vi "Remove Logged Cal.vi"(8 "error in (no error)":errorcluster, 11 "array results in":T1) -> (0 "error out":errorcluster, 2 "update results?":bool, 3 "array results out":T1)   [LabVIEW 2020]
uses:
  Controller Loop/Controller Data.ctl
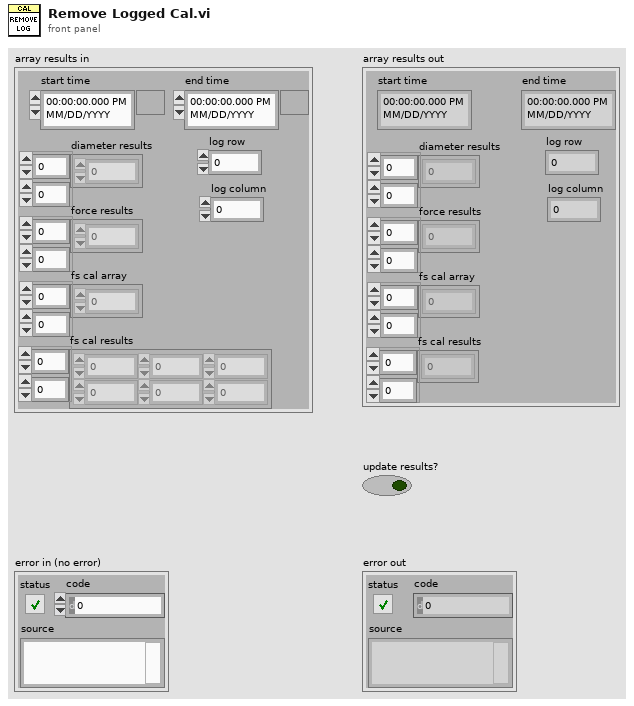
[diagram p1: front panel]
types:
  T1 = typedef "Controller Data.ctl" = cluster{"diameter results":dbl[][], "force results":dbl[][], "fs cal array":dbl[][], "fs cal results":dbl[][], "start time":timestamp, "end time":timestamp, "log row":i32, "log column":i32}
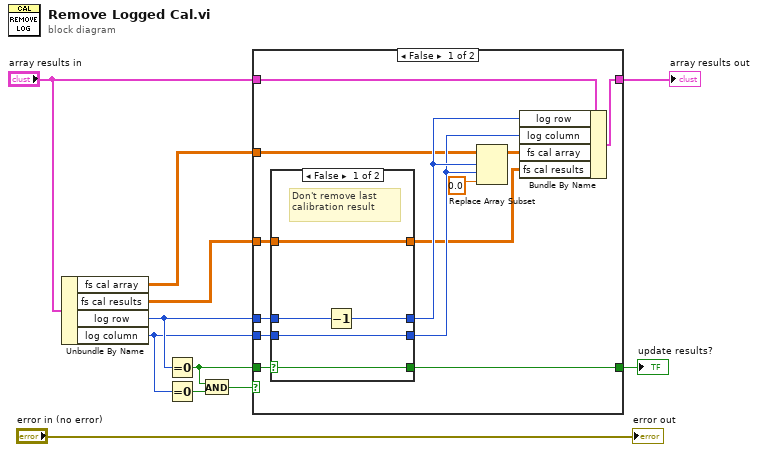
[diagram p0: block diagram]
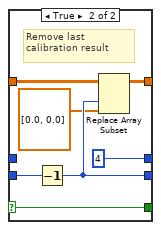
[diagram p2: hidden frame]
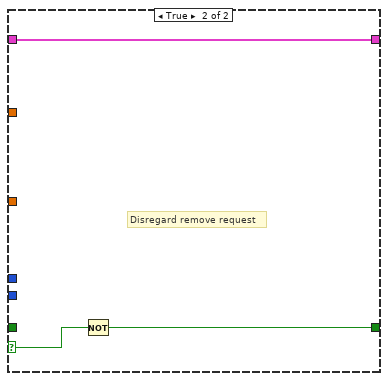
[diagram p3: hidden frame]
diagram:
  n1 = Unbundle By Name("array results in") -> ("fs cal array"=w1:dbl[][], "fs cal results"=w2:dbl[][], "log row"=w4:i32, "log column"=w3:i32)
  n2 = Equal To 0?(x=w4) -> (x = 0?=w6:bool)
  n3 = Equal To 0?(x=w3) -> (x = 0?=w7:bool)
  n4 = And(x=w6, y=w7) -> (x .and. y?=w8:bool)
  n5 = case shown="False" w8 {
    selector: w8 -> [_ w38]
    tunnel: [w19 w39] -> w9
    tunnel: "array results in" -> [w20 w39]
    tunnel: [w16 w37] -> w11
    tunnel: w6 -> [w24 _]
    tunnel: w4 -> [w23 _]
    tunnel: w3 -> [w22 _]
    tunnel: w2 -> [w13 _]
    tunnel: w1 -> [w15 _]
    frame False {
      n6 = case shown="False" w24 {
        selector: w24 -> [w26 w34]
        tunnel: w23 -> [w29 _]
        tunnel: w22 -> [w27 w36]
        tunnel: [w28 4] -> w18
        tunnel: [w27 w31] -> w17
        tunnel: [w26 w34] -> w16
        tunnel: w13 -> [w25 w33]
        tunnel: [w25 w32] -> w12
        frame False {
          # "Don't remove last calibration result"
          n7 = Decrement(x=w29) -> (x-1=w28:i32)
        }
        frame True {
          # "Remove last calibration result"
          n8 = Decrement(x=w36) -> (x-1=w31:i32)
          n9 = Replace Array Subset(array=w33, new element=dbl[] [0.0, 0.0] ("new element/subarray"), index (col)=w31) -> (w32:dbl[][])  [unwired: 1 in]
        }
      }
      n10 = Replace Array Subset(array=w15, new element=0.0 ("new element/subarray"), index (row)=w18, index (col)=w17) -> (w14:dbl[][])
      n11 = Bundle By Name(cluster=w20, "log row"=w18, "log column"=w17, "fs cal array"=w14, "fs cal results"=w12) -> (w19:T1)
    }
    frame True {
      # "Disregard remove request"
      n12 = Not(x=w38) -> (.not. x?=w37:bool)
    }
  }
  "update results?" <- w11
  "array results out" <- w9
  "error out" <- "error in (no error)"
